vi "Get Scan Settings.vi"(11 "Model in":refnum<class "Model.lvclass">) -> (2 "Scan Settings":T1, 3 "Model out":refnum<class "Model.lvclass">)   [LabVIEW 2015, in "Model.lvclass"]
uses:
  Model.lvclass
  Typedefs/ScanSettings.ctl
  Typedefs/FAMT Typedefs.lvlib
  Typedefs/WaveformTypes.ctl
  Typedefs/WaveformSettings.ctl
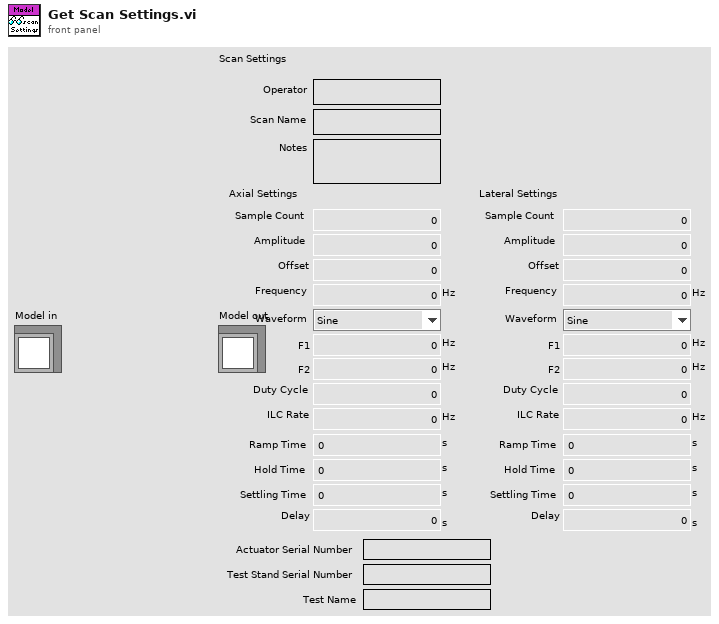
[diagram p1: front panel]
types:
  T1 = typedef "FAMT Typedefs.lvlib/ScanSettings.ctl" = cluster{"Operator":string, "Scan Name":string, "Notes":string, "Axial Settings":T2, "Lateral Settings":T2, "Actuator Serial Number":string, "Test Stand Serial Number":string, "Test Name":string}
  T2 = typedef "FAMT Typedefs.lvlib/WaveformSettings.ctl" = cluster{"Sample Count":u32, "Amplitude":dbl, "Offset":dbl, "Frequency":dbl[unit], "Waveform":T3, "F1":dbl[unit], "F2":dbl[unit], "Duty Cycle":dbl, "ILC Rate":dbl[unit], "Ramp Time":dbl[unit], "Hold Time":dbl[unit], "Settling Time":dbl[unit], "Delay":dbl[unit]}
  T3 = typedef "FAMT Typedefs.lvlib/WaveformTypes.ctl" = enum16{"Sine", "Triangle", "Square", "Sawtooth", "Chirp", "Gaussian", "Trapezoid", "Constant"}
  T4 = typedef "FAMT Typedefs.lvlib/Scan Settings.ctl" = cluster{"Operator":string, "Scan Name":string, "Notes":string, "Axial Settings":T2, "Lateral Settings":T2, "Actuator Serial Number":string, "Actuator Orientation":string, "Actuator Inclination":string, "Test Stand Serial Number":string, "Operating Temperature":string, "Test Name":string}
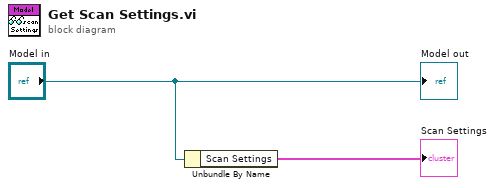
[diagram p0: block diagram]
diagram:
  n1 = Unbundle By Name("Model in") -> ("Scan Settings"=→"Scan Settings":T4)
  "Model out" <- "Model in"
